vi "4155C Get Filename.vi"(3 "error in (no error)":errorcluster) -> (0 "error out":errorcluster, 1 "cancelled":bool, 2 "path":path)   [LabVIEW 2019]
uses:
  4155C Filename.vi
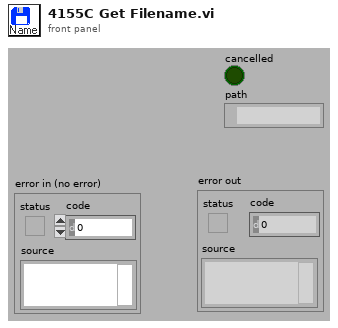
[diagram p1: front panel]
types:
  T1 = enum32{"existing file", "new file", "new or existing file", "existing dir", "new dir", "new or existing dir", "existing file (use LLBs)", "new file (use LLBs)", "new or existing file (use LLBs)", "new or existing file or directory (use LLBs)"}
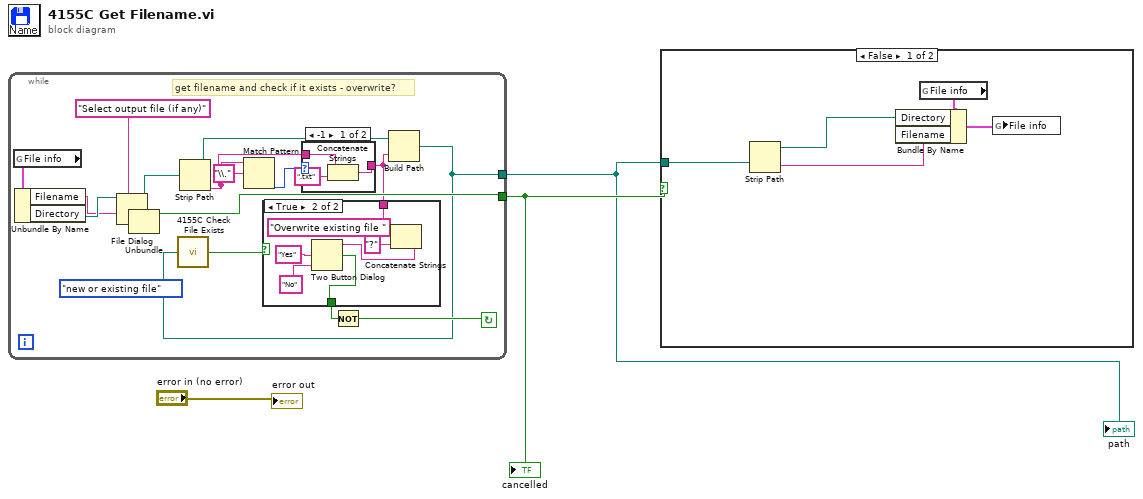
[diagram p0: block diagram]
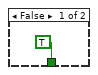
[diagram p3: hidden frame]
diagram:
  n1 = while {
    tunnel: [w8] -> w1
    tunnel: [w17] -> w3
    stop <- w13 continue-if-true
    (unwired) T1."new or existing file" ("select mode (2)")
    # "get filename and check if it exists - overwrite?"
    n2 = global read "4155C Filename.vi" "File info"() -> (w14:cluster{"Filename":string, "Directory":path})
    n3 = Unbundle By Name(w14) -> ("Filename"=w15:string, "Directory"=w16:path)
    n4 = File Dialog(7:"Select output file (if any)" ("prompt"), 9:w15, 11:w16) -> (0:w4:errorcluster, 1:w17:bool, 3:w7:path)  [unwired: 4 in, 1 out]
    n5 = Unbundle(w4) -> ()  [unwired: 3 out]
    n6 = Strip Path(path=w7) -> (stripped path=w6:path, name=w10:string)
    n7 = Match Pattern(string=w10, regular expression="\\.") -> (offset past match=w11:i32)  [unwired: 1 in, 3 out]
    n8 = case shown="-1" w11 {
      tunnel: w10 -> [w20 w23]
      tunnel: [w22 w23] -> w5
      frame -1 {
        n9 = Concatenate Strings(w20, ".txt" ("Substring")) -> (w22:string)
      }
      frame 0, Default {
      }
    }
    n10 = Build Path(base path=w6, name or relative path=w5) -> (appended path=w8:path)
    n11 = call "4155C Check File Exists.vi"("Path"=w8) -> ("Exists?"=w9:bool)
    n12 = case shown="True" w9 {
      tunnel: [TRUE w31] -> w18
      tunnel: w5 -> [_ w28]
      frame False {
      }
      frame True {
        n13 = Concatenate Strings("Overwrite existing file " ("message"), w28, "?" ("Substring")) -> (w26:string)
        n14 = Two Button Dialog(message=w26, 1:"No" ("F button name (\"Cancel\")"), 2:"Yes" ("T button name (\"OK\")")) -> (T button?=w31:bool)
      }
    }
    n15 = Not(x=w18) -> (.not. x?=w13:bool)
  }
  "cancelled" <- w3
  "path" <- w1
  n16 = case shown="False" w3 {
    tunnel: w1 -> [w34 _]
    frame False {
      n17 = Strip Path(path=w34) -> (stripped path=w33:path, name=w32:string)
      n18 = global read "4155C Filename.vi" "File info"() -> (w35:cluster{"Filename":string, "Directory":path})
      n19 = Bundle By Name(cluster=w35, "Directory"=w33, "Filename"=w32) -> (w36:cluster{"Filename":string, "Directory":path})
      n20 = global write "4155C Filename.vi" "File info"(w36) -> ()
    }
    frame True {
    }
  }
  "error out" <- "error in (no error)"
